vi "FileIO-Insert Header Data (string).vi"(0 "path":path, 5 "Field":string="Note", 7 "Data":string, 11 "error in (no error)":errorcluster) -> (4 "path out":path, 15 "error out":errorcluster)   [LabVIEW 2020]
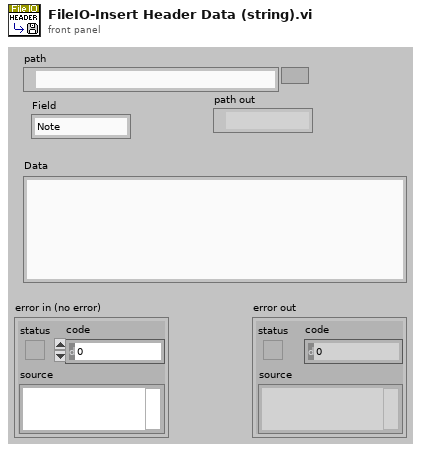
[diagram p1: front panel]
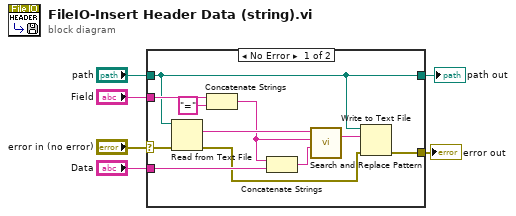
[diagram p0: block diagram]
diagram:
  n1 = case shown="No Error" "error in (no error)" {
    selector: "error in (no error)" -> [w11 w19]
    tunnel: "Data" -> [w16 _]
    tunnel: "path" -> [w7 w18]
    tunnel: [w12 w19] -> w4
    tunnel: "Field" -> [w10 _]
    tunnel: [w7 w18] -> w1
    frame No Error {
      n2 = Read from Text File(file (use dialog)=w7, error in=w11) -> (text=w17:string, error out=w13:errorcluster)  [unwired: 2 in, 2 out]
      n3 = Concatenate Strings(w10, "=" ("string")) -> (w9:string)
      n4 = Concatenate Strings(w9, w16) -> (w15:string)
      n5 = call <vilib>:"Search and Replace Pattern.vi"("string"=w17, "regular expression (\"\")"=w9, "replace string (\"\")"=w15) -> ("result string"=w14:string)  [unwired: 2 in, 1 out]
      n6 = Write to Text File(file (use dialog)=w7, text=w14, error in=w13) -> (error out=w12:errorcluster)  [unwired: 1 in, 2 out]
    }
    frame Error {
    }
  }
  "error out" <- w4
  "path out" <- w1
